vi "StopWrapper.vi"(11 "DLLpath":path) -> ()   [LabVIEW 2014]
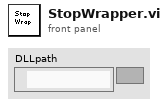
[diagram p1: front panel]
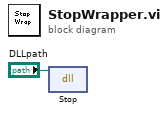
[diagram p0: block diagram]
diagram:
  n1 = dll-call lib="C:/Users/guss2/Desktop/DLLtest/MachineSimulator.dll" fn="Stop"(path in="DLLpath") -> ()  [unwired: 3 in, 2 out]
